vi "Untitled 2 (SubVI).vi"(9 "Haso config file path in":path, 10 "Interaction matrix path in":path, 11 "PathToWavefrontCorrectorSetupFile in":path) -> (0 "CorrectionDataManager out":refnum<class "CorrectionDataManager.lvclass">, 1 "Pupil.lvclass":refnum<class "Pupil.lvclass">, 2 "ModalCoef (new)":refnum<class "ModalCoef.lvclass">, 3 "HasoSlopes out":refnum<class "HasoSlopes.lvclass">, 4 "WavefrontCorrector out":refnum<class "WavefrontCorrector.lvclass">, 5 "radius":sgl, 6 "center":T1, 7 "ComputePhaseSet (new)":refnum<class "ComputePhaseSet.lvclass">)   [LabVIEW 2020]
uses:
  HASO4_3/WaveKit/Classes/WavefrontCorrector/WavefrontCorrector.lvclass
  HASO4_3/WaveKit/Classes/CorrectionDataManager/CorrectionDataManager.lvclass
  HASO4_3/WaveKit/Classes/HasoSlopes/HasoSlopes.lvclass
  HASO4_3/WaveKit/Classes/ComputePhaseSet/ComputePhaseSet.lvclass
  HASO4_3/WaveKit/Classes/Pupil/Pupil.lvclass
  HASO4_3/WaveKit/Classes/ModalCoef/ModalCoef.lvclass
  HASO4_3/WaveKit/Controls/Point2Df.ctl
  HASO4_3/WaveKit/Controls/CircularPupilDetectionParams.ctl
  HASO4_3/WaveKit/Controls/PupilDetectionOption.ctl
  HASO4_3/WaveKit/Controls/CircularAutoDetectionOptions.ctl
  HASO4_3/WaveKit/Controls/PupilDetectionMode.ctl
  HASO4_3/WaveKit/Controls/WavefrontModalReconstructionType.ctl
  HASO4_3/WaveKit/Controls/WavefrontReconstructionMode.ctl
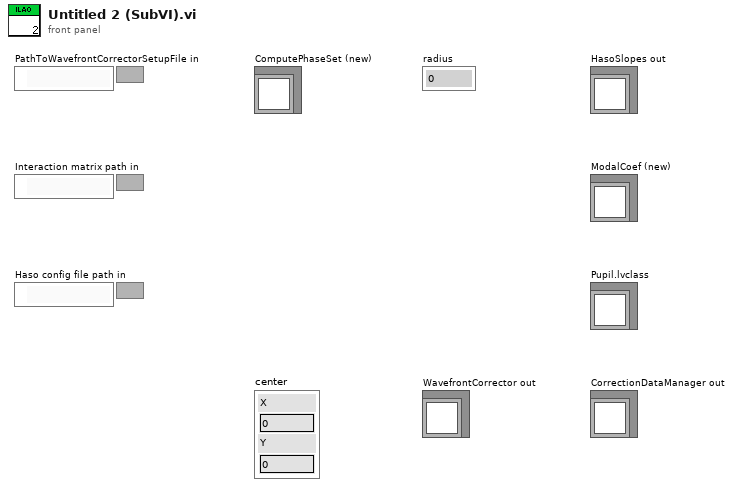
[diagram p1: front panel]
types:
  T1 = typedef "Point2Df.ctl" = cluster{"X":sgl, "Y":sgl}
  T2 = typedef "WavefrontReconstructionMode.ctl" = enum16{"None", "Modal_Legendre", "Modal_Zernike", "Zonal", "Modal_Zonal_Zernike", "Modal_Zonal_Legendre"}
  T3 = typedef "WavefrontModalReconstructionType.ctl" = enum16{"Legendre", "Zernike"}
  T4 = typedef "CircularPupilDetectionParams.ctl" = cluster{"PupilDetectionOption":T5, "AutoDetectionOption":T6, "PupilDetectionMode":T7, "CentralOccultationDetection":bool}
  T5 = typedef "PupilDetectionOption.ctl" = enum16{"Manual", "Automatic"}
  T6 = typedef "CircularAutoDetectionOptions.ctl" = enum16{"manual_radius_auto_center", "manual_center_auto_radius", "auto_radius_auto_center"}
  T7 = typedef "PupilDetectionMode.ctl" = enum16{"inscribed", "circumscribed"}
  T8 = typedef "CasaoManagerGeneralSpecifications.ctl" = cluster{"Wavefront corrector name":string, "Wavefront corrector serial number":string, "Nb actuators":i32, "HASO serial number":string, "Dimension_um":T9}
  T9 = typedef "General dimensions definition.ctl" = cluster{"Size":T10, "Step":T1}
  T10 = typedef "Point2D.ctl" = cluster{"X":u32, "Y":u32}
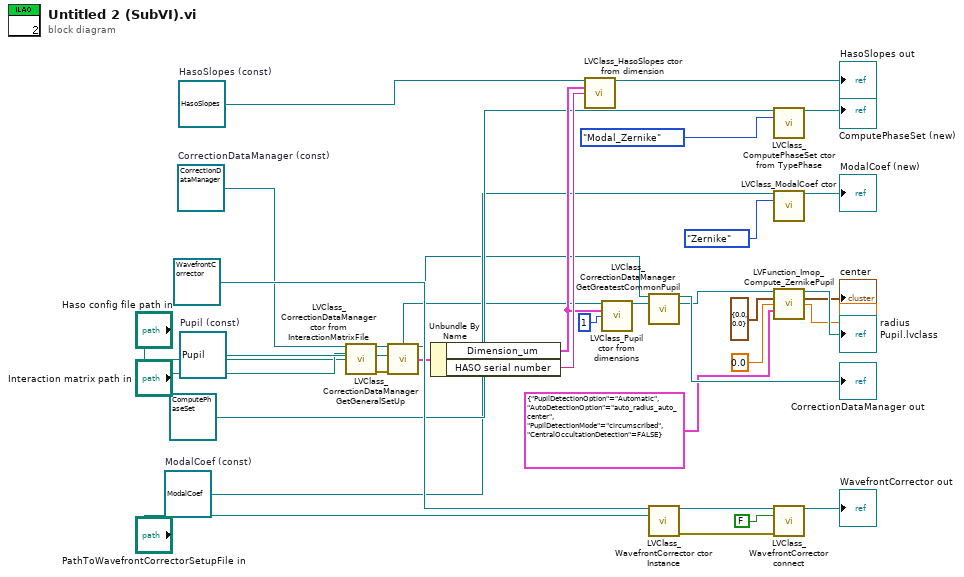
[diagram p0: block diagram]
diagram:
  w23 = refnum<class "HasoSlopes.lvclass"> refnum  # HasoSlopes (const)
  w18 = refnum<class "ModalCoef.lvclass"> refnum  # ModalCoef (const)
  w8 = refnum<class "Pupil.lvclass"> refnum  # Pupil (const)
  w3 = refnum<class "CorrectionDataManager.lvclass"> refnum  # CorrectionDataManager (const)
  n1 = call "LVClass_CorrectionDataManager ctor from InteractionMatrixFile.vi"("CorrectionDataManager (const)"=w3, "Haso config file path"="Haso config file path in", "Interaction matrix path"="Interaction matrix path in") -> ("CorrectionDataManager (new)"=w1:refnum<class "CorrectionDataManager.lvclass">, "error out"=w2:errorcluster)  [unwired: 11 in]
  n2 = call "LVClass_CorrectionDataManager GetGeneralSetUp.vi"("CorrectionDataManager in"=w1, "error in (no error)"=w2) -> ("CorrectionDataManager out"=w7:refnum<class "CorrectionDataManager.lvclass">, "general"=w4:T8)  [unwired: 11 in, 1 out]
  n3 = Unbundle By Name(w4) -> ("Dimension_um"=w24:T9, "HASO serial number"=w25:string)
  n4 = call "LVClass_HasoSlopes ctor from dimension.vi"("HasoSlopes (const)"=w23, "Dimensions_um"=w24, "serial"=w25) -> ("HasoSlopes (new)"=→"HasoSlopes out":refnum<class "HasoSlopes.lvclass">)  [unwired: 11 in, 1 out]
  n5 = call "LVClass_Pupil ctor from dimensions.vi"("Pupil (const)"=w8, "Dimensions_um"=w24, "value"=u8 1) -> ("Pupil (new)"=w10:refnum<class "Pupil.lvclass">)  [unwired: 11 in, 1 out]
  n6 = call "LVClass_CorrectionDataManager GetGreatestCommonPupil.vi"("CorrectionDataManager in"=w7, "Pupil in"=w10) -> ("CorrectionDataManager out"=→"CorrectionDataManager out":refnum<class "CorrectionDataManager.lvclass">, "Pupil out"=w14:refnum<class "Pupil.lvclass">)  [unwired: 11 in, 1 out]
  n7 = call "LVClass_WavefrontCorrector ctor Instance.vi"("WavefrontCorrector (const)"=refnum<class "WavefrontCorrector.lvclass"> refnum ("WavefrontCorrector in"), "PathToWavefrontCorrectorSetupFile"="PathToWavefrontCorrectorSetupFile in") -> ("WavefrontCorrector (new)"=w33:refnum<class "WavefrontCorrector.lvclass">, "error out"=w31:errorcluster)  [unwired: 12 in]
  n8 = call "LVClass_ComputePhaseSet ctor from TypePhase.vi"("ComputePhaseSet (const)"=refnum<class "ComputePhaseSet.lvclass"> refnum ("ComputePhaseSet"), "TypePhase"=WavefrontReconstructionMode."Modal_Zernike") -> ("ComputePhaseSet (new)"=→"ComputePhaseSet (new)":refnum<class "ComputePhaseSet.lvclass">)  [unwired: 12 in, 1 out]
  n9 = call "LVClass_ModalCoef ctor.vi"("ModalCoef (const)"=w18, "TypePhase"=WavefrontModalReconstructionType."Zernike") -> ("ModalCoef (new)"=→"ModalCoef (new)":refnum<class "ModalCoef.lvclass">)  [unwired: 12 in, 1 out]
  n10 = call "LVFunction_Imop_Compute_ZernikePupil.vi"("Pupil.lvclass"=w14, "center in"=T1 {"X"=0.0, "Y"=0.0}, "radius in"=sgl 0.0, "CircularPupilDetectionParams"=T4 {"PupilDetectionOption"=enum."Automatic", "AutoDetectionOption"=enum."auto_radius_auto_center", "PupilDetectionMode"=enum."circumscribed", "CentralOccultationDetection"=FALSE}) -> ("Pupil.lvclass"=→"Pupil.lvclass":refnum<class "Pupil.lvclass">, "center"=→"center":T1, "radius"=→"radius":sgl)  [unwired: 8 in, 1 out]
  n11 = call "LVClass_WavefrontCorrector connect.vi"("WavefrontCorrector in"=w33, "set_init_state_from_config_file"=FALSE, "error in (no error)"=w31) -> ("WavefrontCorrector out"=→"WavefrontCorrector out":refnum<class "WavefrontCorrector.lvclass">)  [unwired: 11 in, 1 out]
